vi "Initialise (Base).vi"(6 "Name":string, 7 "Tick Period [100 ms]":i32=100, 8 "error in (no error)":errorcluster, 10 "Process":refnum<vi>, 11 "Actor in":refnum<class "Actor.lvclass">) -> (0 "error out":errorcluster, 2 "Message Channel":refnum<user-event>, 3 "Actor out":refnum<class "Actor.lvclass">, 5 "Mailbox":refnum<event-registration>)   [LabVIEW 2020, in "Actor.lvclass"]
uses:
  Actor.lvclass
  Message.ctl
  Actor.lvclass/Actor.ctl
  Sequencer/Sequencer.lvclass
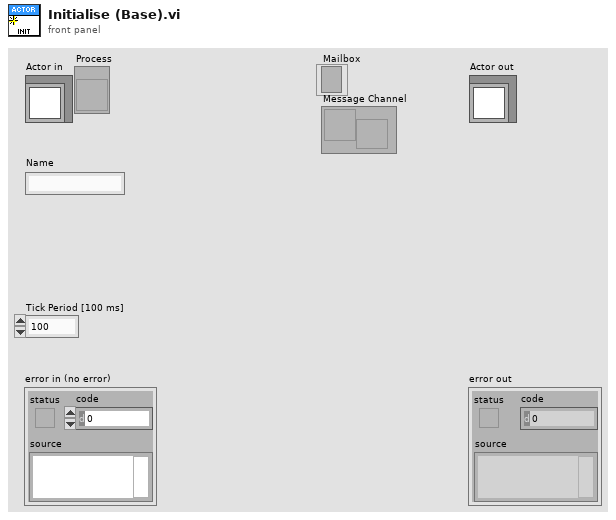
[diagram p1: front panel]
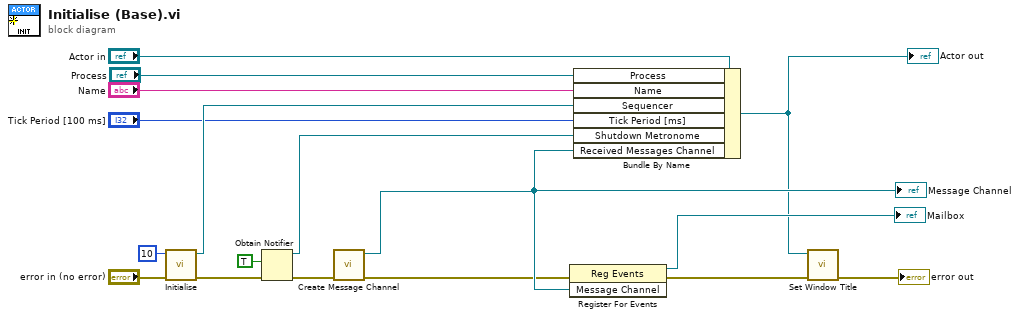
[diagram p0: block diagram]
diagram:
  n1 = call "Initialise.vi"("error in (no error)"="error in (no error)", "Max Steps (10)"=10) -> ("error out"=w5:errorcluster, "Sequencer out"=w14:refnum<class "Sequencer.lvclass">)  [unwired: 8 in]
  n2 = Obtain Notifier(notification data type=TRUE, error in (no error)=w5) -> (notifier out=w11:refnum<notifier>, error out=w9:errorcluster)  [unwired: 2 in, 1 out]
  n3 = call "Create Message Channel.vi"("error in (no error)"=w9) -> ("error out"=w4:errorcluster, "Message Channel"=w6:refnum<user-event>)  [unwired: 9 in]
  "Message Channel" <- w6
  n4 = register-events(error in=w4, w6) -> (reference out=→"Mailbox":refnum<event-registration>, error out=w3:errorcluster)  [unwired: 1 in]
  n5 = Bundle By Name(cluster="Actor in", "Process"="Process", "Name"="Name", "Sequencer"=w14, "Tick Period [ms]"="Tick Period [100 ms]", "Shutdown Metronome"=w11, "Received Messages Channel"=w6) -> (w1:refnum<class "Actor.lvclass">)
  "Actor out" <- w1
  n6 = call "Set Window Title.vi"("error in (no error)"=w3, "Actor in"=w1) -> ("error out"=→"error out":errorcluster)  [unwired: 9 in]
